vi "menu.vi"(8 "Elements":string[](array[string]), 11 "NXT/EV3 2":T1) -> (0 "Goto":dbl, 3 "NXT/EV3":T1)   [LabVIEW 2013]
uses:
  <vilib>/NXT/Subs/LVHSConnector.ctl
  <vilib>/NXT/LegoClasses/BrickReference/BrickReference.lvclass
  <vilib>/NXT/Dual Mode Library/Display/clearDisplay.vi
  <vilib>/NXT/Dual Mode Library/Display/drawPicture.vi
  <vilib>/NXT/Dual Mode Library/Advanced/NXTFlag_Get.vi
  <vilib>/NXT/Dual Mode Library/Advanced/NXTFlag_Clear.vi
  <vilib>/NXT/Dual Mode Library/Waits/Wait_Num.vi
  <vilib>/NXT/Dual Mode Library/Display/drawText_Center.vi
  <vilib>/NXT/Dual Mode Library/Advanced/NXTFlag_Assign.vi
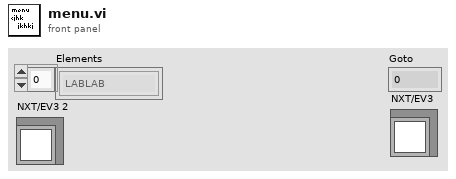
[diagram p1: front panel]
types:
  T1 = typedef "LVHSConnector.ctl" = refnum<class "BrickReference.lvclass">
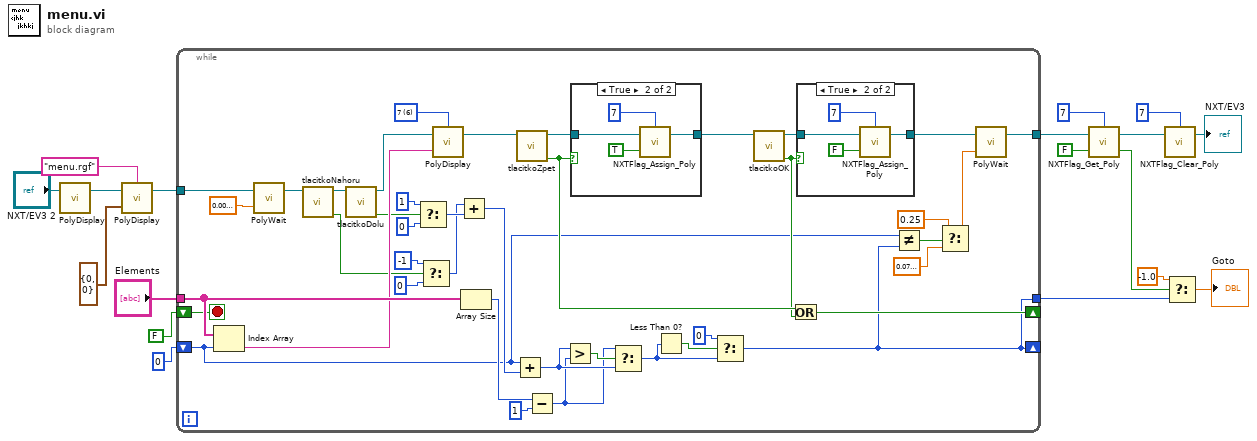
[diagram p0: block diagram]
diagram:
  n1 = call-poly <vilib>:"PolyDisplay.vi"("NXT/EV3"="NXT/EV3 2") -> ("NXT/EV3"=w5:T1)  [unwired: 3 in]
  n2 = call-poly <vilib>:"PolyDisplay.vi"("Origin"=cluster{"X":i16, "Y":i16} {"X"=0, "Y"=0}, "NXT/EV3"=w5, "Filename (*.ric/*.rgf)"="menu.rgf") -> ("NXT/EV3"=w6:T1)  [unwired: 1 in]
  n3 = while {
    shift-right: [w42] -> _
    shift-left: FALSE -> [w43]
    tunnel: "Elements" -> [w46]
    shift-right: [w21] -> _
    shift-left: 0 -> [w20]
    tunnel: [w37] -> w15
    tunnel: [w21] -> w10
    tunnel: w6 -> [w39]
    stop <- w43 stop-if-true
    w44 = i16 6 items=["1", "2", "3", "4", "5", "6", "7", "8", "9", "10", "11", "12"] ("Line")
    n4 = Index Array(array=w46, index=w20) -> (element=w45:string)
    n5 = call-poly <vilib>:"PolyWait.vi"("Time (1 sec)"=sgl 0.01, "NXT/EV3"=w39) -> ("NXT/EV3"=w32:T1)  [unwired: 2 in]
    n6 = call "tlacitkoNahoru.vi"("NXT/EV3"=w32) -> ("Boolean"=w36:bool, "NXT/EV3 2"=w30:T1)  [unwired: 9 in]
    n7 = call "tlacitkoDolu.vi"("NXT/EV3"=w30) -> ("Boolean"=w33:bool, "NXT/EV3 2"=w31:T1)  [unwired: 9 in]
    n8 = Select(t=1, s=w33, f=0) -> (s? t:f=w54:i32)
    n9 = Select(t=-1, s=w36, f=0) -> (s? t:f=w53:i32)
    n10 = call-poly <vilib>:"PolyDisplay.vi"("Text"=w45, "NXT/EV3"=w31, "Line"=w44) -> ("NXT/EV3"=w27:T1)  [unwired: 1 in]
    n11 = Add(x=w53, y=w54) -> (x+y=w52:i32)
    n12 = Array Size(array=w46) -> (size(s)=w59:i32)
    n13 = Add(x=w20, y=w52) -> (x+y=w50:i32)
    n14 = call "tlacitkoZpet.vi"("NXT/EV3"=w27) -> ("Boolean"=w35:bool, "NXT/EV3 2"=w26:T1)  [unwired: 9 in]
    n15 = Subtract(x=w59, y=1) -> (x-y=w25:i32)
    n16 = Greater?(x=w50, y=w25) -> (0:w51:bool)
    n17 = case shown="True" w35 {
      tunnel: w26 -> [w65 w67]
      tunnel: [w65 w66] -> w29
      frame False {
      }
      frame True {
        n18 = call-poly <vilib>:"NXTFlag_Assign_Poly.vi"("Flag State"=TRUE, "NXT/EV3"=w67, "NXT/EV3 Flag Number"=i8 7) -> ("NXT/EV3"=w66:T1)  [unwired: 1 in]
      }
    }
    n19 = Select(t=w25, s=w51, f=w50) -> (s? t:f=w48:i32)
    n20 = Less Than 0?(x=w48) -> (x < 0?=w49:bool)
    n21 = Select(t=0, s=w49, f=w48) -> (s? t:f=w21:i32)
    n22 = call "tlacitkoOK.vi"("NXT/EV3"=w29) -> ("Boolean"=w34:bool, "NXT/EV3 2"=w28:T1)  [unwired: 9 in]
    n23 = Or(x=w35, y=w34) -> (x .or. y?=w42:bool)
    n24 = case shown="True" w34 {
      tunnel: w28 -> [w60 w62]
      tunnel: [w60 w61] -> w38
      frame False {
      }
      frame True {
        n25 = call-poly <vilib>:"NXTFlag_Assign_Poly.vi"("Flag State"=FALSE, "NXT/EV3"=w62, "NXT/EV3 Flag Number"=i8 7) -> ("NXT/EV3"=w61:T1)  [unwired: 1 in]
      }
    }
    n26 = Not Equal?(x=w20, y=w21) -> (x != y?=w24:bool)
    n27 = Select(t=sgl 0.25, s=w24, f=sgl 0.08 ("Time (1 sec)")) -> (s? t:f=w22:sgl)
    n28 = call-poly <vilib>:"PolyWait.vi"("Time (1 sec)"=w22, "NXT/EV3"=w38) -> ("NXT/EV3"=w37:T1)  [unwired: 2 in]
  }
  n29 = call-poly <vilib>:"NXTFlag_Get_Poly.vi"("Clear if Found"=FALSE, "NXT/EV3"=w15, "NXT/EV3 Flag Number"=7) -> ("status"=w12:bool, "NXT/EV3"=w8:T1)
  n30 = call-poly <vilib>:"NXTFlag_Clear_Poly.vi"("NXT/EV3"=w8, "NXT/EV3 Flag Number"=7) -> ("NXT/EV3"=→"NXT/EV3":T1)  [unwired: 2 in]
  n31 = Select(t=-1.0, s=w12, f=w10) -> (s? t:f=→"Goto":dbl)
